vi "GMLAN DisableNormalCommunication.vi"(8 "error in (no error)":errorcluster, 10 "Parameter":T1, 11 "diag ref in":T2) -> (0 "error out":errorcluster, 1 "success?":bool, 3 "diag ref out":T2)   [LabVIEW 2013, in "GMLAN.lvlib"]
uses:
  GMLAN.lvlib
  <vilib>/Automotive Diagnostic Command Set/Diagnostic Transport.llb/Diag Reference.ctl
  <vilib>/Automotive Diagnostic Command Set/Diagnostic Transport.llb/Transport Protocol Selector.ctl
  <vilib>/Automotive Diagnostic Command Set/Diagnostic Transport.llb/Diag CAN Frame Log.ctl
  _SubVIs/DisableNormalCommunication_Parameter.ctl
  <vilib>/Automotive Diagnostic Command Set/Diagnostic Transport.llb/Apply Diagnostic Error.vi
  <vilib>/Automotive Diagnostic Command Set/Diagnostic Transport.llb/Diag Globals.vi
  <vilib>/Automotive Diagnostic Command Set/Diagnostic Transport.llb/Diagnostic Service Send.vi
  <vilib>/Automotive Diagnostic Command Set/Diagnostic Transport.llb/Diagnostic Response Recv.vi
  <vilib>/addons/Automotive Diagnostic Command Set/NI_Automotive Diagnostic Command Set.lvlib
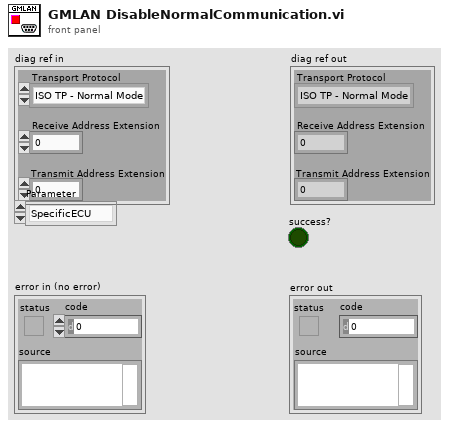
[diagram p1: front panel]
types:
  T1 = typedef "GMLAN.lvlib/DisableNormalCommunication_Parameter.ctl" = enum8{"SpecificECU", "EntireNetwork"}
  T2 = typedef "NI_Automotive Diagnostic Command Set.lvlib/Diag Reference.ctl" = cluster{"Diag CAN Handle":u32, "Transport Protocol":T3, "Receive Address Extension":u8, "Transmit Address Extension":u8, "Receive CAN Id":u32, "Transmit CAN Id":u32, "Diag CAN Queue":refnum<queue>, "Log Frames ?":bool, "My TP Address":u8, "Other TP Address":u8, "T1":u16, "T2":u16, "T3":u16, "T4":u16, "Tx SN":u8, "Block Size":u8, "Rx SN":u8, "VW TP Initialized?":bool, "Tx block no":u8, "baud rate":u32, "Interface":string, "Channel Diag CAN Handle":u32, "UDP Connection ID":refnum<k16>, "TCP Connection ID":refnum<k5>, "Target IP Addr":u32, "Source Address":u16, "Target Address":u16, "Send Header NACK?":bool, "DLL Handle":u32, "NAD":u8, "Time Stamp read first":dbl, "Time Stamp read last":dbl, "Time Stamp write first":dbl, "Time Stamp write last":dbl, "Time Stamp write":dbl, "Time Stamp read":dbl}
  T3 = typedef "NI_Automotive Diagnostic Command Set.lvlib/Transport Protocol Selector.ctl" = enum16{"ISO TP - Normal Mode", "ISO TP - Mixed Mode", "VW TP 2.0", "Diagnostics on IP", "ISO TP LIN"}
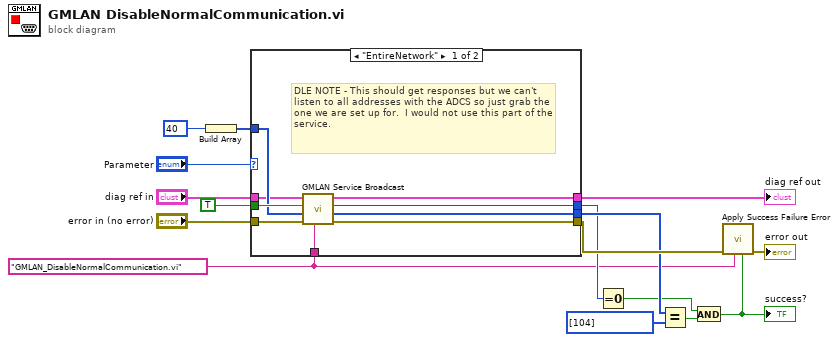
[diagram p0: block diagram]
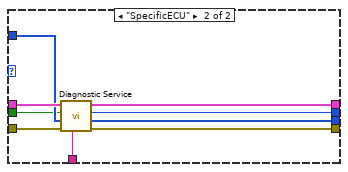
[diagram p2: hidden frame]
diagram:
  w6 = "GMLAN_DisableNormalCommunication.vi" ("error source")
  n1 = Build Array(u8 40) -> (w10:u8[])
  n2 = case shown="\"EntireNetwork\"" "Parameter" {
    tunnel: "error in (no error)" -> [w25 w34]
    tunnel: [w20 w33] -> w15
    tunnel: [w19 w32] -> w14
    tunnel: [w17 w31] -> w13
    tunnel: "diag ref in" -> [w22 w30]
    tunnel: w10 -> [w23 w29]
    tunnel: [w18 w28] -> w9
    tunnel: w6 -> [w21 w27]
    tunnel: TRUE ("require response?") -> [w24 w26]
    frame "EntireNetwork" {
      # "DLE NOTE - This should get responses but we can't listen to all addresses with the ADCS so just grab the one we are set up for.  I would not use this part of the service."
      n3 = call "GMLAN Service Broadcast.vi"("error source"=w21, "error in (no error)"=w25, "data in"=w23, "require response?"=w24, "diag ref in"=w22) -> ("error out"=w20:errorcluster, "data out"=w19:u8[], "error code"=w18:u8, "diag ref out"=w17:T2)  [unwired: 3 in]
    }
    frame "SpecificECU" {
      n4 = call <vilib>:"Diagnostic Service.vi"("error source"=w27, "error in (no error)"=w34, "data in"=w29, "require response?"=w26, "diag ref in"=w30) -> ("error out"=w33:errorcluster, "data out"=w32:u8[], "error code"=w28:u8, "diag ref out"=w31:T2)  [unwired: 1 in, 2 out]
    }
  }
  "diag ref out" <- w13
  n5 = Equal To 0?(x=w9) -> (x = 0?=w3:bool)
  n6 = Equal?(x=w14, y=u8[] [104]) -> (x = y?=w4:bool)
  n7 = And(x=w3, y=w4) -> (x .and. y?=w7:bool)
  "success?" <- w7
  n8 = call <vilib>:"Apply Success Failure Error.vi"("success code"=w7, "error source"=w6, "error in (no error)"=w15) -> ("error out"=→"error out":errorcluster)  [unwired: 8 out]
